vi "End Regular Cleaning Service.vi"(11 "Hotel":string) -> ()   [LabVIEW 2023]
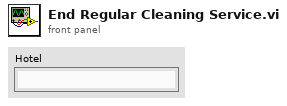
[diagram p1: front panel]
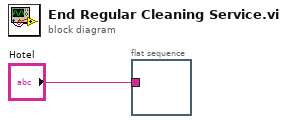
[diagram p0: block diagram]
diagram:
  n1 = flat-sequence {
    tunnel: "Hotel" -> [_]
    frame #0 {
    }
  }
